vi "Start Sync.vi"(8 "error in (no error)":errorcluster, 11 "gRPC Server in":refnum<class "Ex1_server.lvclass">) -> (0 "error out":errorcluster, 3 "gRPC Server out":refnum<class "Ex1_server.lvclass">)   [LabVIEW 2019, in "Ex1_server.lvlib" / "Ex1_server.lvclass"]
uses:
  Ex1_server.lvclass
  Ex1_server.lvclass/Ex1_server.ctl
  TemperatureSensor/TemperatureSensor.lvclass
  RPC Messages/Temperature/Temperature_Data.ctl
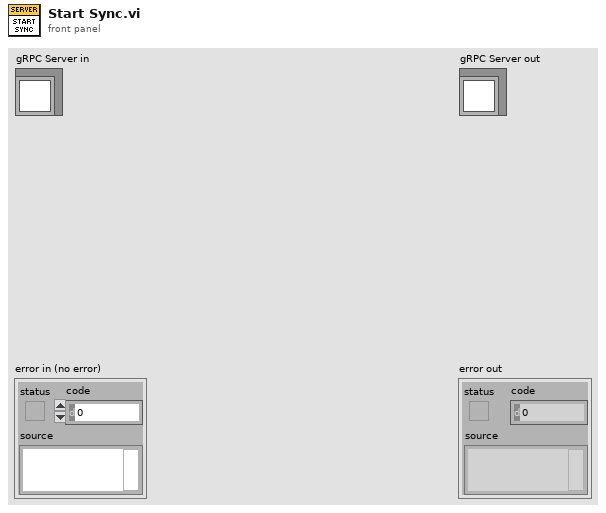
[diagram p1: front panel]
types:
  T1 = typedef "Ex1_server.lvlib/Ex1_server.lvclass/Temperature_Data.ctl" = cluster{"temperature":dbl}
  T2 = typedef "Ex1_server.lvlib/Ex1_server.lvclass/Server gRPC UEs.ctl" = cluster{"TemperatureService_Measure gRPC UE":refnum<user-event>}
  T3 = typedef "gprc-lvsupport-release.lvlib/grpcId.ctl" = u64
  T4 = typedef "Ex1_server.lvlib/Ex1_server.lvclass/Units_Data.ctl" = cluster{"unit":i32}
  T5 = typedef "Ex1_server.lvlib/Ex1_server.lvclass/Server State Data.ctl" = cluster{"sensor":refnum<class "TemperatureSensor.lvclass">}
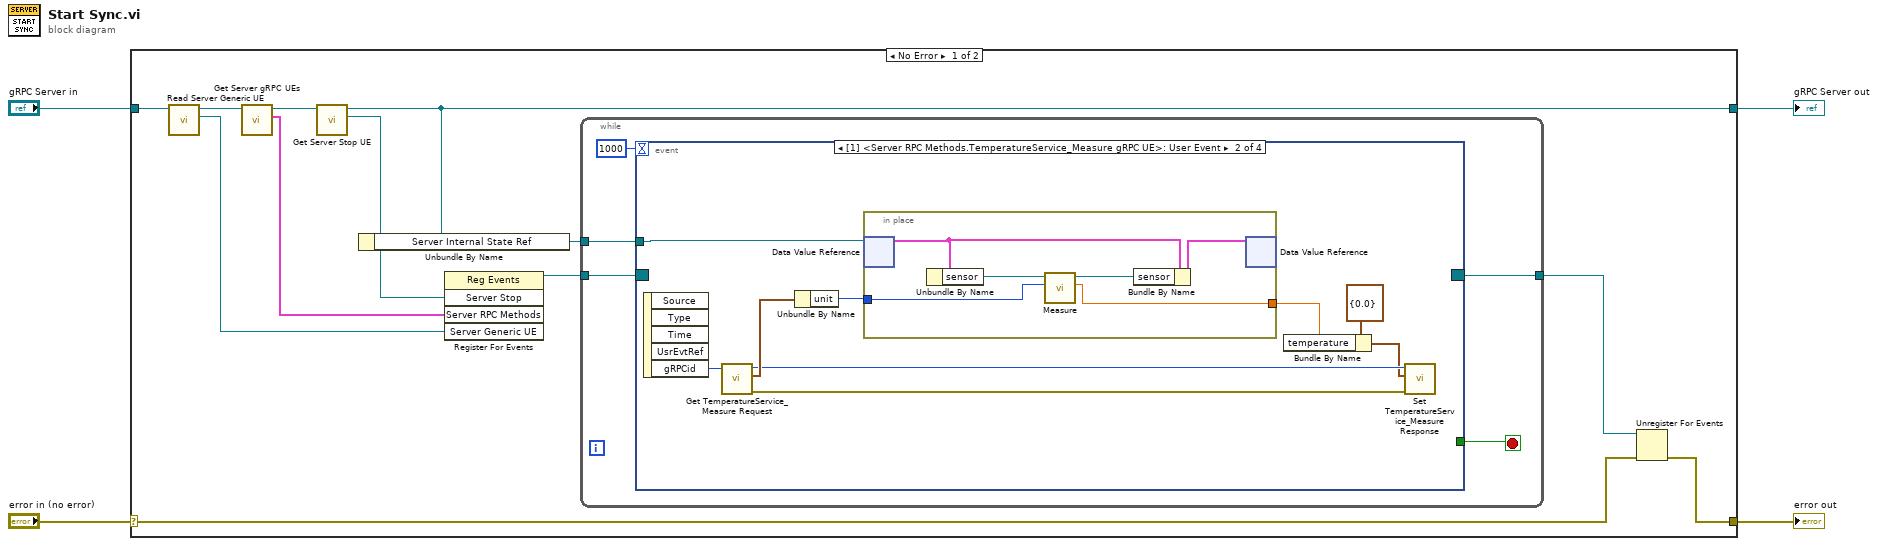
[diagram p0: block diagram]
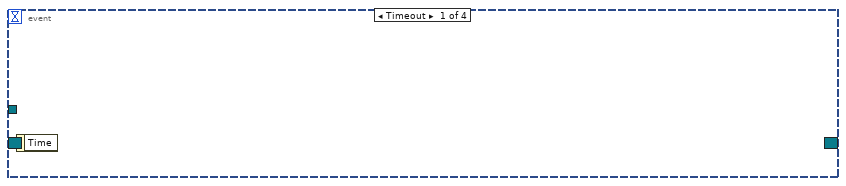
[diagram p2: hidden frame]
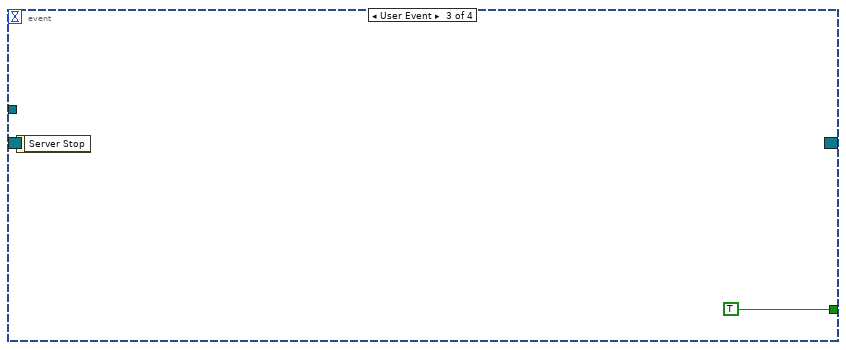
[diagram p3: hidden frame]
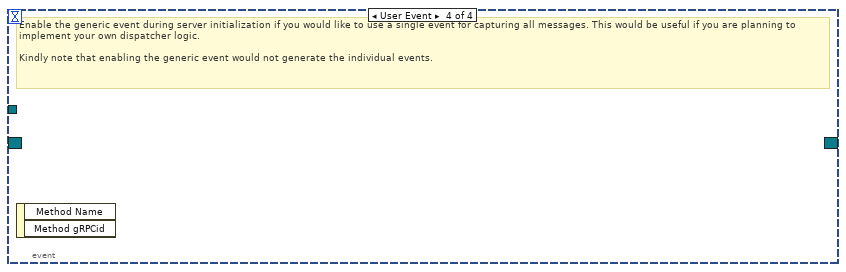
[diagram p4: hidden frame]
diagram:
  n1 = case shown="No Error" "error in (no error)" {
    selector: "error in (no error)" -> [w11 w39]
    tunnel: [w10 w39] -> w3
    tunnel: [w6 w38] -> w1
    tunnel: "gRPC Server in" -> [w9 w38]
    frame No Error {
      n2 = call "Read Server Generic UE.vi"("Template Server in"=w9) -> ("Server Generic UE"=w7:refnum<user-event>, "Template Server out"=w8:refnum<class "Ex1_server.lvclass">)  [unwired: 9 in]
      n3 = call "Get Server gRPC UEs.vi"("OOP Server in"=w8) -> ("Server RPC Methods"=w14:T2, "OOP Server out"=w16:refnum<class "Ex1_server.lvclass">)  [unwired: 9 in]
      n4 = call "Get Server Stop UE.vi"("OOP Server in"=w16) -> ("Server Stop"=w15:refnum<user-event>, "OOP Server out"=w6:refnum<class "Ex1_server.lvclass">)  [unwired: 9 in]
      n5 = Unbundle By Name(w6) -> ("Server Internal State Ref"=w5:refnum<data-value>)
      n6 = register-events(w15, w14, w7) -> (reference out=w13:refnum<event-registration>)  [unwired: 2 in, 1 out]
      n7 = while {
        tunnel: w13 -> [w21]
        tunnel: [w19] -> w12
        tunnel: w5 -> [w17]
        stop <- w20 stop-if-true
        n8 = event "RPC Methods Event Structure" shown="[1] <Server RPC Methods.TemperatureService_Measure gRPC UE>: User Event" {
          selector: w21 -> [_ _ _ _]
          dyn-events: [_ _ _ _] -> w19
          timeout: 1000 -> [_ _ _ _]
          tunnel: [_ _ TRUE _] -> w20
          tunnel: w17 -> [_ w30 _ _]
          event Timeout {
            n9 = event-data() -> ()  [unwired: 1 in, 1 out]
          }
          event User Event {
            n10 = event-data() -> ("gRPCid"=w29:T3)  [unwired: 1 in, 4 out]
            n11 = call "Get TemperatureService_Measure Request.vi"("gRPCid in"=w29) -> ("error out"=w22:errorcluster, "Message Data"=w28:T4, "gRPCid out"=w26:T3)  [unwired: 8 in]
            n12 = Unbundle By Name(w28) -> ("unit"=w27:i32)
            n13 = in-place {
              in-place-border: w27 -> [w32]
              in-place-border: [w31] -> w24
              n14 = in-place-dvr #1(w30) -> (w35:T5)  [unwired: 1 out]
              n15 = Unbundle By Name(w35) -> ("sensor"=w36:refnum<class "TemperatureSensor.lvclass">)
              n16 = call "Measure.vi"("unit"=w32, "TemperatureSensor in"=w36) -> ("measurement"=w31:dbl, "TemperatureSensor out"=w33:refnum<class "TemperatureSensor.lvclass">)  [unwired: 7 in, 1 out]
              n17 = Bundle By Name(cluster=w35, "sensor"=w33) -> (w34:T5)
              n18 = in-place-dvr #1(w34) -> ()  [unwired: 2 out]
            }
            n19 = Bundle By Name(cluster=T1 {"temperature"=0.0} ("Message Data"), "temperature"=w24) -> (w23:T1)
            n20 = call "Set TemperatureService_Measure Response.vi"("error in (no error)"=w22, "Message Data"=w23, "gRPCid in"=w26) -> ()  [unwired: 8 in, 1 out]
          }
          event User Event {
            n21 = event-data() -> ()  [unwired: 1 in, 1 out]
          }
          event User Event {
            # "Enable the generic event during server initialization if you would like to use a single event for capturing all messages. This would be useful if you are planning to implement your own dispatcher logic. \n\nKindly note that enabling the generic event would not generate the individual events."
            n22 = event-data() -> ()  [unwired: 1 in, 2 out]
          }
        }
      }
      n23 = Unregister For Events(event registration refnum=w12, error in=w11) -> (error out=w10:errorcluster)
    }
    frame Error {
    }
  }
  "error out" <- w3
  "gRPC Server out" <- w1
